vi "Read Public Events.vi"(8 "error in (no error)":errorcluster, 11 "TCPConnectionHandler in":refnum<class "ConnectionHandler.lvclass">) -> (0 "error out":errorcluster, 2 "Connection Handler Public Events":T1, 3 "TCPConnectionHandler out":refnum<class "ConnectionHandler.lvclass">)   [LabVIEW 2013, in "MQTT Server.lvlib" / "ConnectionHandler.lvclass"]
uses:
  ConnectionHandler.lvclass
  Public Events -- Cluster.ctl
  ConnectionHandler.lvclass/ConnectionHandler.ctl
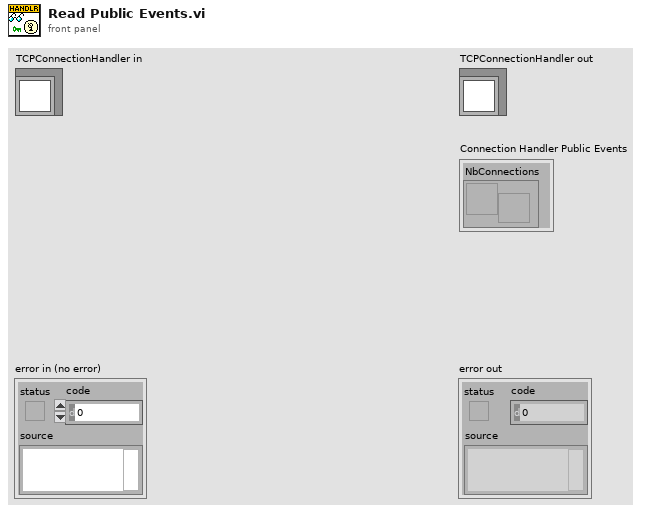
[diagram p1: front panel]
types:
  T1 = typedef "MQTT Server.lvlib/ConnectionHandler.lvclass/Public Events -- Cluster.ctl" = cluster{"NbConnections":refnum<user-event>}
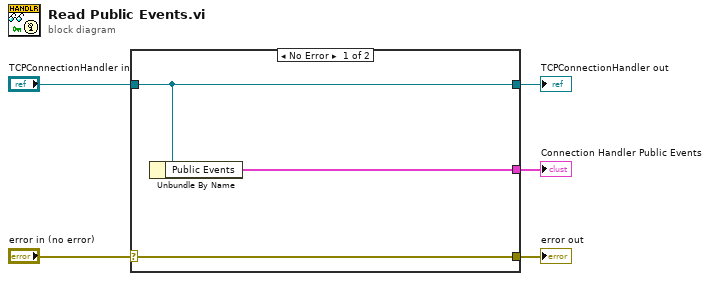
[diagram p0: block diagram]
diagram:
  n1 = case shown="No Error" "error in (no error)" {
    selector: "error in (no error)" -> [w8 w9]
    tunnel: [w8 w9] -> w4
    tunnel: [w7 w10] -> w2
    tunnel: "TCPConnectionHandler in" -> [w7 w10]
    tunnel: [w6 _] -> w1
    frame No Error {
      n2 = Unbundle By Name(w7) -> ("Public Events"=w6:T1)
    }
    frame Error {
    }
  }
  "error out" <- w4
  "TCPConnectionHandler out" <- w2
  "Connection Handler Public Events" <- w1
